vi "GT_LoadExtConfig.vi"(1 "pFileName":string, 2 "rtn_In":cluster{"rtn":i16, "Func":string}) -> (0 "rtn_Out":cluster{"rtn":i16, "Func":string})   [LabVIEW 2014]
uses:
  data/data/ExtMdl.dll
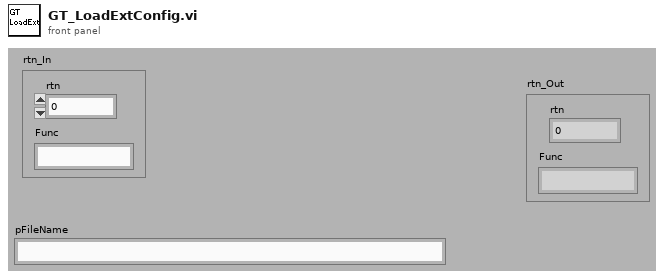
[diagram p1: front panel]
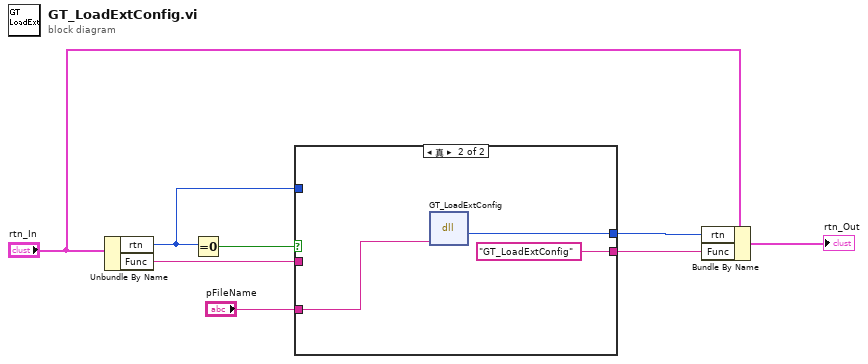
[diagram p0: block diagram]
diagram:
  n1 = Unbundle By Name("rtn_In") -> ("rtn"=w2:i16, "Func"=w7:string)
  n2 = Equal To 0?(x=w2) -> (x = 0?=w8:bool)
  n3 = case shown="真" w8 {
    tunnel: w7 -> [w9 _]
    tunnel: [w10 w13] -> w4
    tunnel: [w9 "GT_LoadExtConfig" ("Func")] -> w3
    tunnel: w2 -> [w10 _]
    tunnel: "pFileName" -> [_ w11]
    frame False {
    }
    frame True {
      n4 = dll-call lib="PTH2Iabs DNewGTS AC-800LWin7版源程序-20170926datadata\nExtMdl.dll" fn="GT_LoadExtConfig"("pFileName"=w11) -> ("rtn"=w13:i16)  [unwired: 4 in, 2 out]
    }
  }
  n5 = Bundle By Name(cluster="rtn_In", "rtn"=w4, "Func"=w3) -> (→"rtn_Out":cluster{"rtn":i16, "Func":string})
